vi "clearDisplay.vi"(8 "error in (no error)":errorcluster, 11 "StaticOutputEditor in":refnum<class "StaticOutputEditor.lvclass">) -> (0 "error out":errorcluster, 3 "StaticOutputEditor out":refnum<class "StaticOutputEditor.lvclass">)   [LabVIEW 2011, in "Views.lvlib" / "ScriptEditor.lvlib" / "StaticOutputEditor.lvclass"]
uses:
  StaticOutputEditor.lvclass
  StaticOutputEditor.lvclass/StaticOutputEditor.ctl
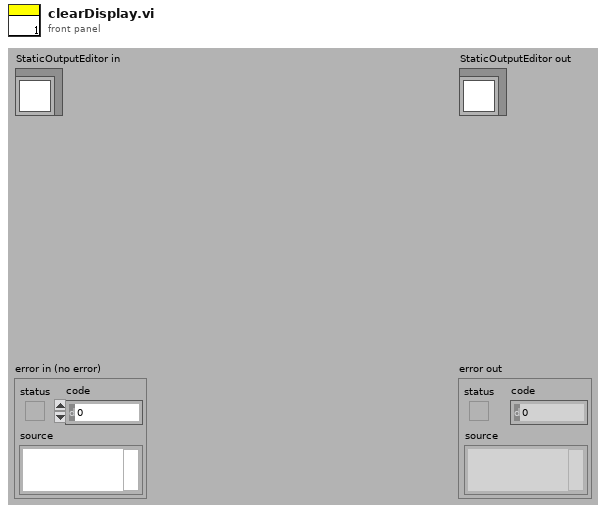
[diagram p1: front panel]
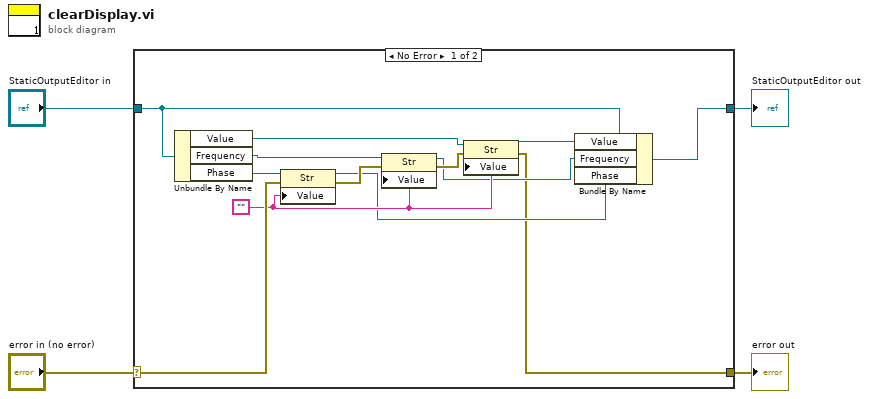
[diagram p0: block diagram]
diagram:
  n1 = case shown="No Error" "error in (no error)" {
    selector: "error in (no error)" -> [w16 w19]
    tunnel: [w5 w19] -> w3
    tunnel: [w6 w18] -> w1
    tunnel: "StaticOutputEditor in" -> [w7 w18]
    frame No Error {
      w11 = ""
      n2 = Unbundle By Name(w7) -> ("Value"=w13:refnum<vi>, "Frequency"=w15:refnum<vi>, "Phase"=w17:refnum<vi>)
      n3 = property class="Str"(reference=w17, error in=w16, "Value"=w11) -> (reference out=w8:refnum<vi>, error out=w14:errorcluster)
      n4 = property class="Str"(reference=w15, error in=w14, "Value"=w11) -> (reference out=w9:refnum<vi>, error out=w12:errorcluster)
      n5 = property class="Str"(reference=w13, error in=w12, "Value"=w11) -> (reference out=w10:refnum<vi>, error out=w5:errorcluster)
      n6 = Bundle By Name(cluster=w7, "Value"=w10, "Frequency"=w9, "Phase"=w8) -> (w6:refnum<class "StaticOutputEditor.lvclass">)
    }
    frame Error {
    }
  }
  "error out" <- w3
  "StaticOutputEditor out" <- w1
